vi "Update Current Temperature.vi"(8 "error in (no error)":errorcluster, 10 "Current Temperature":dbl, 11 "Cooler UI in":refnum<class "Programmatic Controller.lvclass">) -> (0 "error out":errorcluster, 3 "Cooler UI out":refnum<class "Programmatic Controller.lvclass">)   [LabVIEW 2018, in "Programmatic Controller.lvclass"]
doc: "Update the log with a report of the new temperature."
uses:
  Programmatic Controller.lvclass
  Programmatic Controller.lvclass/Programmatic Controller.ctl
panel:
  in  "New indoor temperature":string="New indoor temperature: %f\\n"
  in  "Initial indoor temperature":string="Initial indoor temperature: %f\\n"
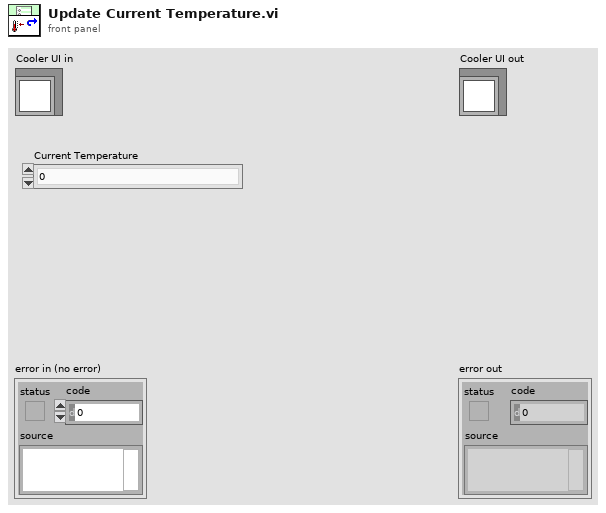
[diagram p1: front panel]
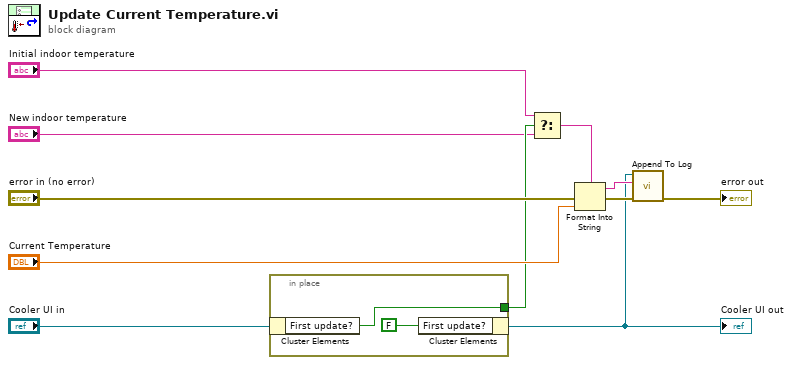
[diagram p0: block diagram]
diagram:
  n1 = in-place {
    in-place-border: [w12] -> w3
    n2 = in-place-cluster #1("Cooler UI in") -> ("First update?"=w12:bool)
    n3 = in-place-cluster #1("First update?"=FALSE) -> (w4:refnum<class "Programmatic Controller.lvclass">)
  }
  "Cooler UI out" <- w4
  n4 = Select(t="Initial indoor temperature", s=w3, f="New indoor temperature") -> (s? t:f=w6:string)
  n5 = Format Into String(format string=w6, error in="error in (no error)", "Current Temperature") -> (resulting string=w11:string, error out=w10:errorcluster)  [unwired: 1 in]
  n6 = call "Append To Log.vi"("error in (no error)"=w10, "String"=w11, "Cooler Alternate UI in"=w4) -> ("error out"=→"error out":errorcluster)  [unwired: 8 in]
